vi "correct image perspective.vi"(7 "error in":errorcluster) -> (27 "error out":errorcluster)   [LabVIEW 2020]
panel:
  in  "Image To Correct":path=path "C:/Users/musahim/Downloads/f3m5c.png"
  out "Image In":T1(plugin-control)
  in  "Calibration File Path":path=path "C:/Users/musahim/Downloads/f3m5c cali.png"
  out "Image Out":T1(plugin-control)
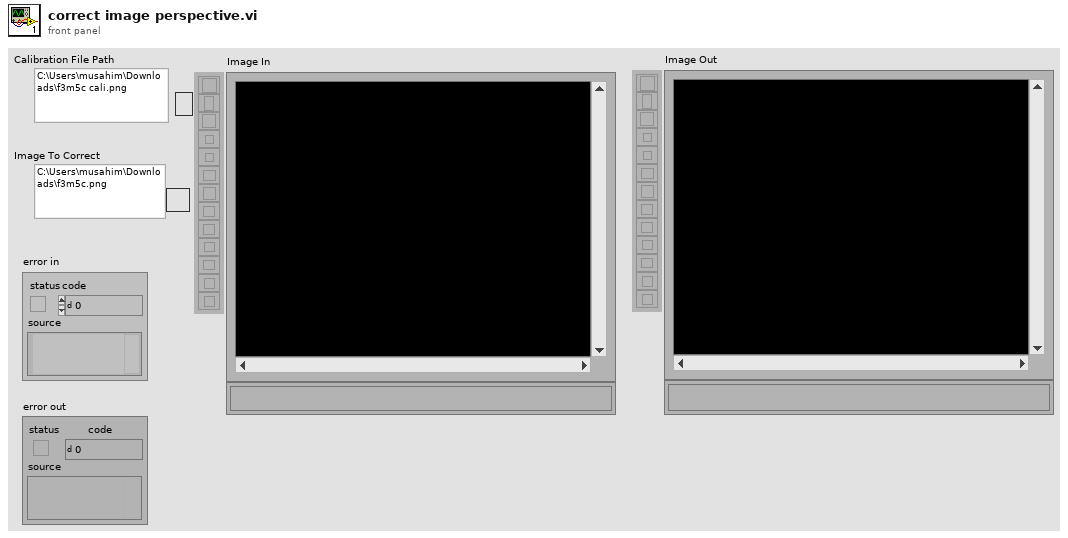
[diagram p1: front panel]
types:
  T1 = typedef "IMAQ Image.ctl" = refnum<image>
  T2 = typedef "Image Type" = u32
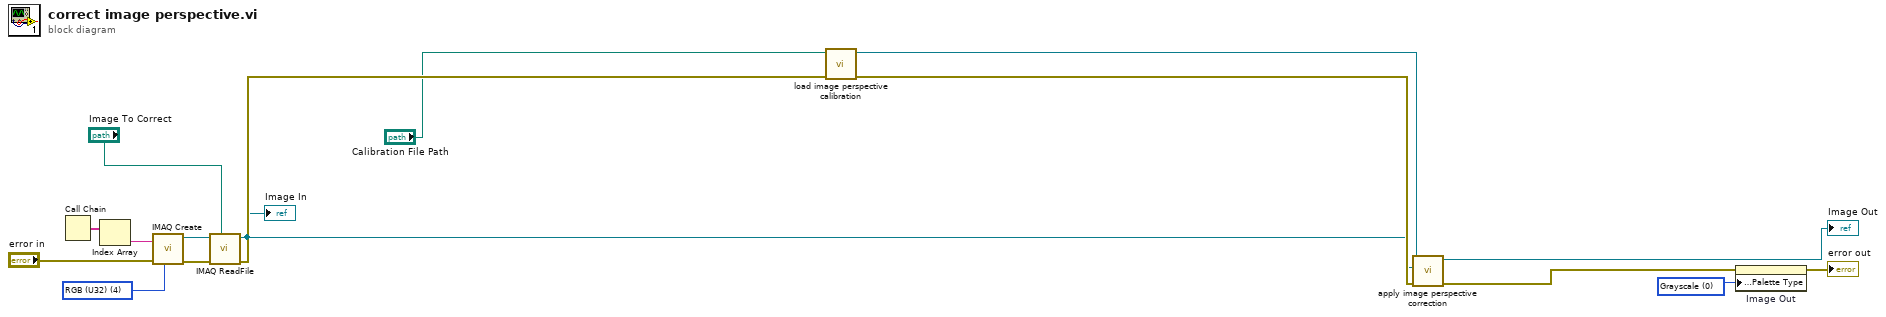
[diagram p0: block diagram]
diagram:
  w3 = u32 0 items=["Grayscale", "Binary", "Gradient", "Rainbow", "Temperature", "User Defined", "Binary 16 Bit", "Gradient 16 Bit", "Rainbow 16 Bit", "Temperature 16 Bit", "User Defined 16 Bit"] ("Palette Type")
  w10 = T2 4 items=["Grayscale (U8)", "Grayscale (I16)", "Grayscale (SGL)", "Complex (CSG)", "RGB (U32)", "HSL (U32)", "RGB (U64)", "Grayscale (U16)"] ("Image Type")
  n1 = Call Chain() -> (call chain=w12:string[])
  n2 = Index Array(array=w12) -> (element=w11:string)  [unwired: 1 in]
  n3 = call "IMAQ Create"("Image Name"=w11, "Image Type"=w10, "error in (no error)"="error in") -> ("New Image"=w15:T1, "error out"=w14:errorcluster)  [unwired: 1 in, 1 out]
  n4 = call "IMAQ ReadFile"("File Path"="Image To Correct", "error in (no error)"=w14, "Image"=w15) -> ("error out"=w16:errorcluster, "Image Out"=w2:T1)  [unwired: 2 in, 5 out]
  "Image In" <- w2
  n5 = call "load image perspective calibration.vi"("error in (no error)"=w16, "Calibration File Path"="Calibration File Path") -> ("error out"=w7:errorcluster, "Refnum out"=w8:T1)  [unwired: 8 in]
  n6 = call "apply image perspective correction.vi"("error in (no error)"=w7, "Calibration Image"=w2, "Image To Correct"=w8) -> ("error out"=w6:errorcluster, "Corrected Image"=→"Image Out":T1)  [unwired: 7 in]
  n7 = property on="Image Out" class="ImageControl"(error in=w6, "Palette:Palette Type"=w3) -> (error out=→"error out":errorcluster)  [unwired: 1 in, 1 out]
